vi "Initialize.vi"(7 "Custom Device Name":string, 8 "error in":errorcluster, 9 "Compiled Settings":variant, 10 "Custom Device API in":refnum<class "Custom Device API.lvclass">, 11 "Custom Device in":refnum<class "SystemMonitor Engine.lvclass">) -> (0 "error out":errorcluster, 3 "Custom Device out":refnum<class "SystemMonitor Engine.lvclass">)   [LabVIEW 2026, in "SystemMonitor Engine.lvlib" / "SystemMonitor Engine.lvclass"]
uses:
  SystemMonitor Engine.lvclass
  <userlib>/Custom Device Interfaces_v1.lvlibp/CustomDeviceAPI/Custom Device API.lvclass
  Types/TargetSettings.ctl
  SystemMonitor Engine.lvclass/SystemMonitor Engine.ctl
  Processes/Template.Async.vi
  Logging/Utilities/Log.Error.vi
  <userlib>/NIVS Inline Async API (Express)/_VS Inline Async API (Express)/VS Inline Async API (Express)/VS Inline Async API (Express).lvclass
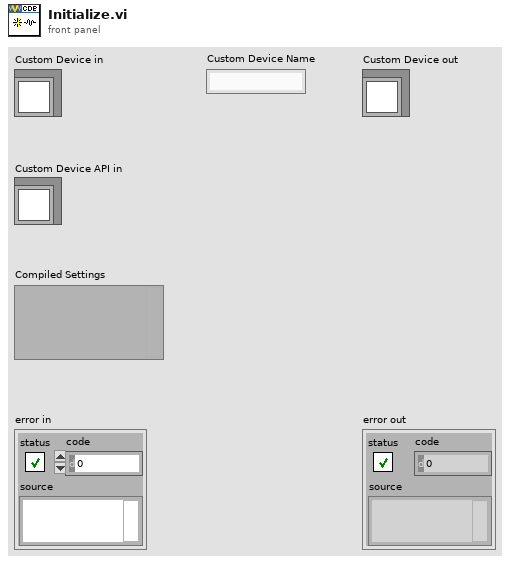
[diagram p1: front panel]
types:
  T1 = typedef "SystemMonitor Engine.lvlib/SystemMonitor Engine.lvclass/TargetSettings.ctl" = cluster{"Update Rate (Hz)":dbl, "# of CPU Cores":i32}
  T2 = typedef "GroupedChannelRefs.ctl" = cluster{"Read":cluster{"Refs":cluster{"Data Reference":i32, "Offset":u64, "Length":u64}[], "Values":dbl[]}[], "Write":cluster{"Refs":cluster{"Data Reference":i32, "Offset":u64, "Length":u64}[], "Values":dbl[]}[], "ReadWrite":cluster{"Refs":i32[], "Values":dbl[], "Reset Values":dbl[]}[], "LUT":variant}
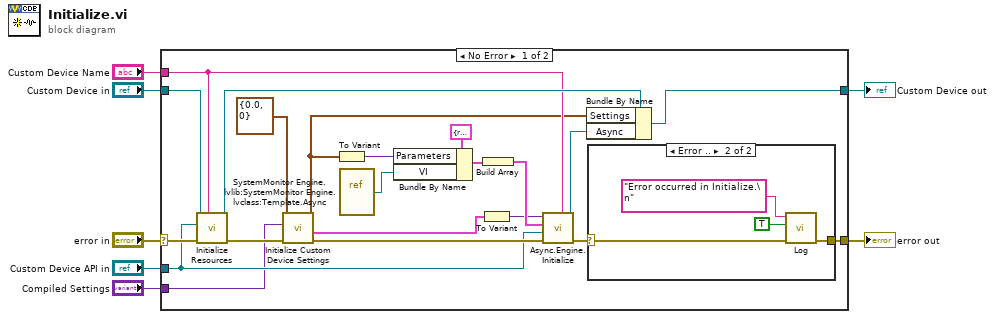
[diagram p0: block diagram]
diagram:
  n1 = case shown="No Error" "error in" {
    selector: "error in" -> [w28 w35]
    tunnel: "Custom Device in" -> [w15 w34]
    tunnel: "Custom Device API in" -> [w12 _]
    tunnel: [w23 w34] -> w3
    tunnel: [w26 w35] -> w6
    tunnel: "Compiled Settings" -> [w9 _]
    tunnel: "Custom Device Name" -> [w16 _]
    frame No Error {
      n2 = call "Initialize Resources.vi"("Custom Device Name"=w16, "error in"=w28, "Custom Device API in"=w12, "Custom Device in"=w15) -> ("error out"=w25:errorcluster, "Custom Device out"=w21:refnum<class "SystemMonitor Engine.lvclass">)  [unwired: 6 in]
      n3 = call "Initialize Custom Device Settings.vi"("error in"=w25, "Compiled Settings"=w9, "Engine Settings in"=T1 {"Update Rate (Hz)"=0.0, "# of CPU Cores"=0} ("Settings")) -> ("error out"=w24:errorcluster, "ChannelRefs"=w8:T2, "Engine Settings out"=w11:T1)  [unwired: 6 in]
      n4 = To Variant(anything=w11) -> (Variant=w14:variant)
      n5 = vi-ref "SystemMonitor Engine.lvlib:SystemMonitor Engine.lvclass:Template.Async.vi"() -> (w22:refnum<vi>)
      n6 = Bundle By Name(cluster=cluster{"VI":refnum<vi>, "Parameters":variant} {"VI"=refnum, "Parameters"=variant} ("Process"), "Parameters"=w14, "VI"=w22) -> (w19:cluster{"VI":refnum<vi>, "Parameters":variant})
      n7 = To Variant(anything=w8) -> (Variant=w13:variant)
      n8 = Build Array(w19) -> (w18:cluster{"VI":refnum<vi>, "Parameters":variant}[])
      n9 = call <userlib>:"Async.Engine.Initialize.vi"("Custom Device Name"=w16, "error in"=w24, "Custom Device API in"=w12, "Processes"=w18, "Compiled.InlineAsync.Settings"=w13) -> ("error out"=w27:errorcluster, "Async out"=w17:refnum<class "VS Inline Async API (Express).lvclass">)  [unwired: 5 in]
      n10 = Bundle By Name(cluster=w21, "Settings"=w11, "Async"=w17) -> (w23:refnum<class "SystemMonitor Engine.lvclass">)
      n11 = case shown="Error .." w27 {
        selector: w27 -> [w29 w32]
        tunnel: [w29 w31] -> w26
        frame No Error {
        }
        frame Error {
          n12 = call-poly "Log.vi"("error in"=w32, "Add to log file? (F)"=TRUE, "Message"="Error occurred in Initialize.\n") -> ("error out"=w31:errorcluster)  [unwired: 8 in]
        }
      }
    }
    frame Error {
    }
  }
  "error out" <- w6
  "Custom Device out" <- w3
